vi "Eurotherm - Front Panel - Simple x 2.vi"() -> ()   [LabVIEW 2011]
uses:
  Common/Utilities/VI Control/Control - Display State.ctl
panel:
  out "Message":string
  in  "Set 2":bool
  in  "Required Setpoint 2":dbl min=-10.0 max=10.0 format="%.3f"
  out "Setpoint 2":dbl format="%.3f"
  out "Temperature 2":dbl caption="Dummy 2" format="%.3f"
  in  "Set 1":bool
  in  "Required Setpoint 1":dbl min=-10.0 max=10.0 format="%.3f"
  out "Setpoint 1":dbl format="%.3f"
  out "Temperature 1":dbl caption="Dummy 1" format="%.3f"
  out "Activity":bool
  in  "Exit":bool
  out "Error":errorcluster
  # "Eurotherm Temperature Controller"
  # "Controller 1"
  # "Controller 2"
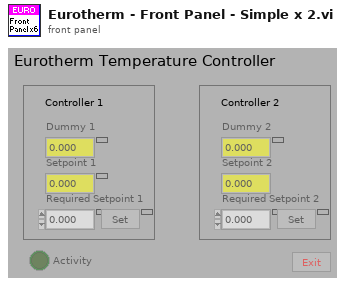
[diagram p1: front panel]
types:
  T1 = typedef "Control - Display State.ctl" = enum16{"Enabled", "Disabled", "Disabled and Grayed"}
  T2 = typedef "Eurotherm - Setups.ctl" = T3[]
  T3 = typedef "Eurotherm - Setup.ctl" = cluster{"Communication":T4, "Name":string, "Enable":bool, "Max Set Point":dbl, "Min Set Point":dbl, "Units":string, "Graph Data":u32, "Sensor type":T8, "Calibration File Path":path, "Conversion Type":T9}
  T4 = typedef "Eurotherm - Communication.ctl" = cluster{"Com Port":T5, "Address":T6, "Baud Rate":T7}
  T5 = typedef "Com Port - Numeric.ctl" = i32
  T6 = typedef "Eurotherm - Address.ctl" = u8
  T7 = typedef "Com Port - Baud Rate.ctl" = u32
  T8 = typedef "Sensors - Temperature Sensor Type.ctl" = enum16{"RhFe", "Pt", "K type thermocouple", "W5 type thermocouple", "No Conversion"}
  T9 = typedef "Sensors - Conversion Type.ctl" = enum16{"Linear", "Spline"}
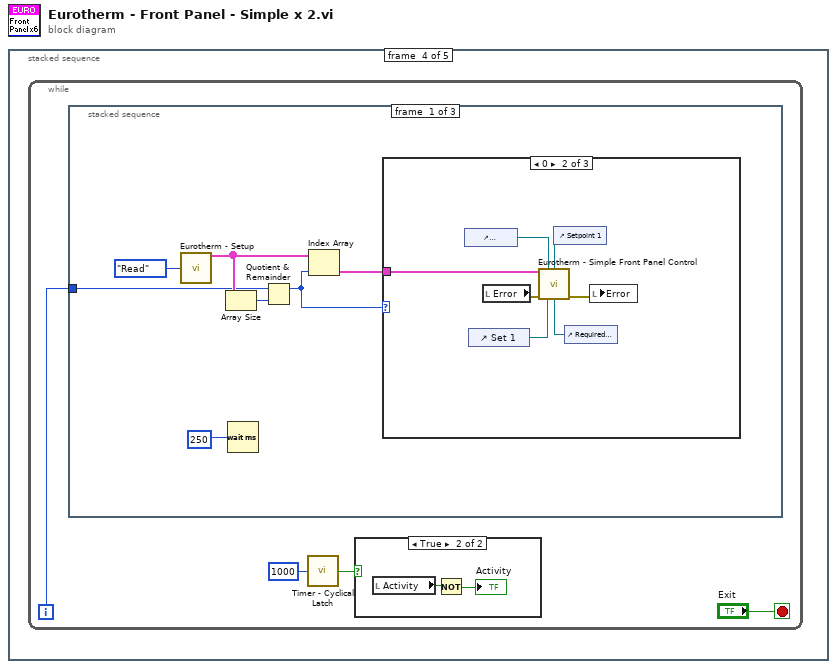
[diagram p0: block diagram]
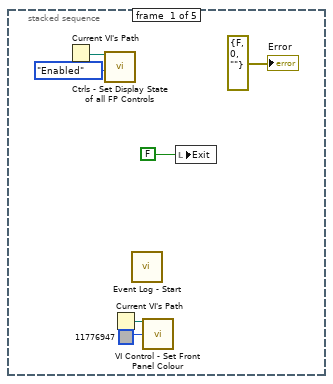
[diagram p2: hidden frame]
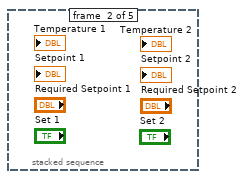
[diagram p3: hidden frame]
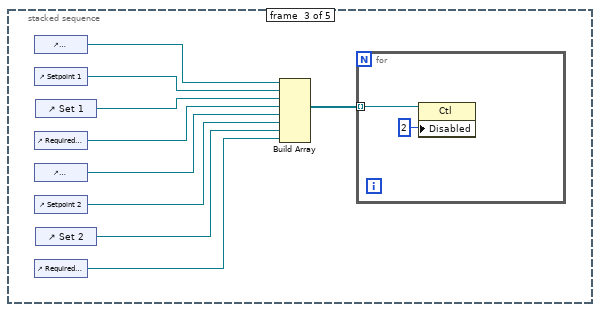
[diagram p4: hidden frame]
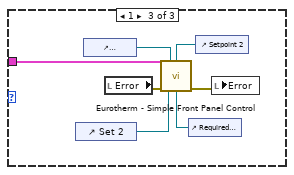
[diagram p6: hidden frame]
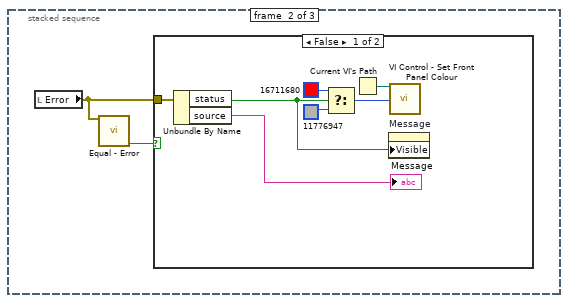
[diagram p7: hidden frame]
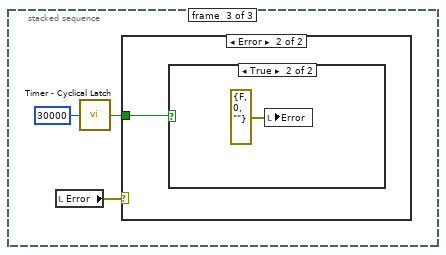
[diagram p9: hidden frame]
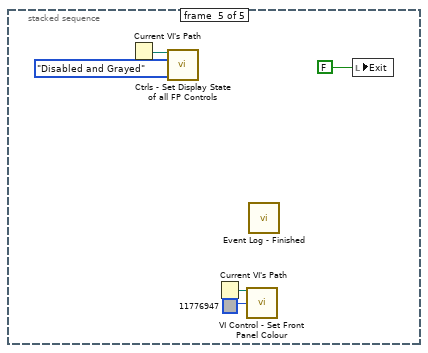
[diagram p13: hidden frame]
diagram:
  n1 = stacked-sequence {
    frame #0 {
      n2 = Current VI's Path() -> (path=w6:path)
      n3 = call "Ctrls - Set Display State of all FP Controls.vi"("VI Path"=w6, "Display State"=Control_-_Display_State."Enabled") -> ()  [unwired: 18 in]
      n4 = Current VI's Path() -> (path=w1:path)
      n5 = call "Event Log - Start.vi"() -> ()  [unwired: 1 in]
      n6 = call "VI Control - Set Front Panel Colour.vi"("VI Path"=w1, "Front Panel Colour"=u32 11776947) -> ()  [unwired: 13 in, 1 out]
      n7 = local write "Exit"(FALSE) -> ()
      "Error" <- errorcluster {"status"=FALSE, "code"=0, "source"=""} ("Error")
    }
    frame #1 {
    }
    frame #2 {
      n8 = control-ref of="Temperature 1"() -> (w15:refnum<vi>)
      n9 = control-ref of="Setpoint 1"() -> (w14:refnum<vi>)
      n10 = control-ref of="Required Setpoint 1"() -> (w12:refnum<vi>)
      n11 = control-ref of="Temperature 2"() -> (w11:refnum<vi>)
      n12 = control-ref of="Setpoint 2"() -> (w9:refnum<vi>)
      n13 = control-ref of="Required Setpoint 2"() -> (w7:refnum<vi>)
      n14 = control-ref of="Set 1"() -> (w13:refnum<vi>)
      n15 = control-ref of="Set 2"() -> (w8:refnum<vi>)
      n16 = Build Array(w15, w14, w13, w12, w11, w9, w8, w7) -> (w10:refnum<vi>[])
      n17 = for {
        tunnel: w10 -> [w17] mode=indexing
        n18 = property class="Ctl"(reference=w17, "Disabled"=u8 2) -> ()  [unwired: 1 in, 2 out]
      }
    }
    frame #3 {
      n19 = while {
        i -> [w18]
        stop <- "Exit" stop-if-true
        n20 = stacked-sequence {
          tunnel: w18 -> [w25 _ _]
          frame #0 {
            n21 = call "Eurotherm - Setup.vi"("Action"=enum16{"Read", "Write"}."Read") -> ("Setup Out"=w26:T2)  [unwired: 12 in, 2 out]
            n22 = Array Size(array=w26) -> (size(s)=w27:i32)
            n23 = Wait (ms)(milliseconds to wait=u32 250) -> ()  [unwired: 1 out]
            n24 = Quotient & Remainder(x=w25, y=w27) -> (x-y*floor(x/y)=w23:i32)  [unwired: 1 out]
            n25 = Index Array(array=w26, index=w23) -> (element=w24:T3)
            n26 = case shown="0" w23 {
              tunnel: w24 -> [_ w35 w36]
              frame Default {
              }
              frame 0 {
                n27 = control-ref of="Temperature 1"() -> (w34:refnum<vi>)
                n28 = control-ref of="Set 1"() -> (w31:refnum<vi>)
                n29 = local read "Error"() -> (w29:errorcluster)
                n30 = control-ref of="Setpoint 1"() -> (w33:refnum<vi>)
                n31 = control-ref of="Required Setpoint 1"() -> (w32:refnum<vi>)
                n32 = call "Eurotherm - Simple Front Panel Control.vi"("Setup"=w35, "Temperature"=w34, "Setpoint"=w33, "error in (no error)"=w29, "Set"=w31, "Required Setpoint"=w32) -> ("error out"=w30:errorcluster)  [unwired: 9 in]
                n33 = local write "Error"(w30) -> ()
              }
              frame 1 {
                n34 = control-ref of="Set 2"() -> (w38:refnum<vi>)
                n35 = control-ref of="Temperature 2"() -> (w40:refnum<vi>)
                n36 = local read "Error"() -> (w41:errorcluster)
                n37 = control-ref of="Required Setpoint 2"() -> (w37:refnum<vi>)
                n38 = control-ref of="Setpoint 2"() -> (w39:refnum<vi>)
                n39 = call "Eurotherm - Simple Front Panel Control.vi"("Setup"=w36, "Temperature"=w40, "Setpoint"=w39, "error in (no error)"=w41, "Set"=w38, "Required Setpoint"=w37) -> ("error out"=w42:errorcluster)  [unwired: 9 in]
                n40 = local write "Error"(w42) -> ()
              }
            }
          }
          frame #1 {
            n41 = local read "Error"() -> (w44:errorcluster)
            n42 = call "Equal - Error.vi"("Value In"=w44) -> ("Equal to previous value"=w43:bool)  [unwired: 13 in, 1 out]
            n43 = case shown="False" w43 {
              tunnel: w44 -> [w47 _]
              frame False {
                n44 = Unbundle By Name(w47) -> ("status"=w46:bool, "source"=→"Message":string)
                n45 = Select(t=u32 16711680, s=w46, f=u32 11776947) -> (s? t:f=w48:u32)
                n46 = Current VI's Path() -> (path=w51:path)
                n47 = property on="Message" class="Str"("Visible"=w46) -> ()  [unwired: 2 in, 2 out]
                n48 = call "VI Control - Set Front Panel Colour.vi"("VI Path"=w51, "Front Panel Colour"=w48) -> ()  [unwired: 13 in, 1 out]
              }
              frame True {
              }
            }
          }
          frame #2 {
            n49 = local read "Error"() -> (w53:errorcluster)
            n50 = call "Timer - Cyclical Latch.vi"("Timer (msec)"=u32 30000) -> ("Timer Trigger"=w52:bool)  [unwired: 14 in]
            n51 = case shown="Error" w53 {
              tunnel: w52 -> [_ w55]
              frame No Error {
              }
              frame Error {
                n52 = case shown="True" w55 {
                  frame False {
                  }
                  frame True {
                    n53 = local write "Error"(errorcluster {"status"=FALSE, "code"=0, "source"=""} ("Error")) -> ()
                  }
                }
              }
            }
          }
        }
        n54 = call "Timer - Cyclical Latch.vi"("Timer (msec)"=u32 1000) -> ("Timer Trigger"=w20:bool)  [unwired: 14 in]
        n55 = case shown="True" w20 {
          frame False {
          }
          frame True {
            n56 = local read "Activity"() -> (w57:bool)
            n57 = Not(x=w57) -> (.not. x?=→"Activity":bool)
          }
        }
      }
    }
    frame #4 {
      n58 = Current VI's Path() -> (path=w62:path)
      n59 = call "Ctrls - Set Display State of all FP Controls.vi"("VI Path"=w62, "Display State"=Control_-_Display_State."Disabled and Grayed") -> ()  [unwired: 18 in]
      n60 = Current VI's Path() -> (path=w60:path)
      n61 = call "VI Control - Set Front Panel Colour.vi"("VI Path"=w60, "Front Panel Colour"=u32 11776947) -> ()  [unwired: 13 in, 1 out]
      n62 = call "Event Log - Finished.vi"() -> ()  [unwired: 1 in]
      n63 = local write "Exit"(FALSE) -> ()
    }
  }
